vi "Write Settings File.vi"(8 "error in (no error)":errorcluster, 11 "Settings":T1={"LCR VISA Resource"="", "PSU VISA Resource"="", "AI Task"="AI_Task", "AO Task"="AO_Task", "DO Task"="DO_Task", "Report Directory"=path ""}) -> (0 "error out":errorcluster)   [LabVIEW 2018]
uses:
  controls/Settings.ctl
  d75c569a-e9c5-441d-9376-d96455150058.vi
  <vilib>/JDP Science/JSONtext/Variant to JSON Text.vi
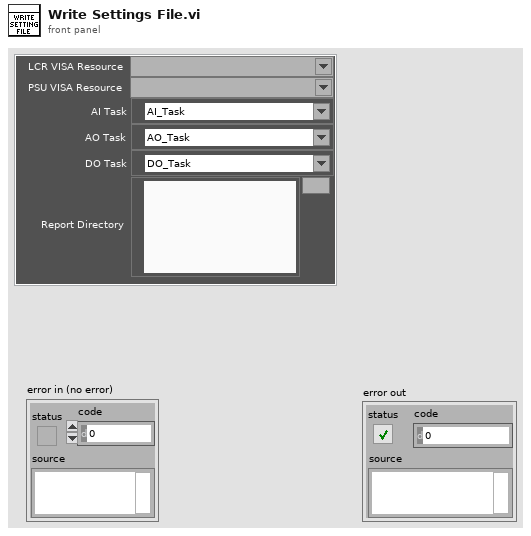
[diagram p1: front panel]
types:
  T1 = typedef "Settings.ctl" = cluster{"LCR VISA Resource":refnum<visa-resource-name>, "PSU VISA Resource":refnum<visa-resource-name>, "AI Task":refnum<k21>, "AO Task":refnum<k21>, "DO Task":refnum<k21>, "Report Directory":path}
  T2 = enum16{"open", "replace", "create", "open or create", "replace or create", "replace or create with confirmation"}
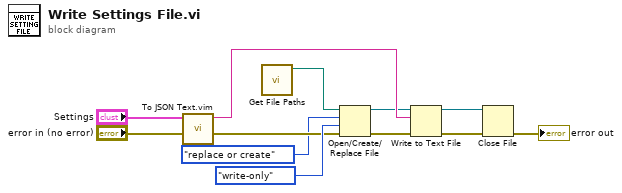
[diagram p0: block diagram]
diagram:
  n1 = call "To JSON Text.vim"("error in (no error)"="error in (no error)", "Anything"="Settings") -> ("error out"=w9:errorcluster, "<JSON>"=w6:string)  [unwired: 8 in]
  n2 = call "Get File Paths.vi"() -> ("Settings Path"=w12:path)  [unwired: 10 in, 1 out]
  n3 = Open/Create/Replace File(file path (use dialog)=w12, error in=w9, operation (0:open)=T2."replace or create", access (0:read/write)=enum16{"read/write", "read-only", "write-only"}."write-only") -> (refnum out=w5:refnum<file>, error out=w7:errorcluster)  [unwired: 2 in, 1 out]
  n4 = Write to Text File(file (use dialog)=w5, text=w6, error in=w7) -> (refnum out=w3:refnum<file>, error out=w4:errorcluster)  [unwired: 1 in, 1 out]
  n5 = Close File(refnum=w3, error in=w4) -> (error out=→"error out":errorcluster)  [unwired: 1 out]
